vi "CallEdit.vi"(9 "Self Enqueuer":refnum<class "Message Enqueuer.lvclass">, 10 "Configuration":refnum<data-value>, 11 "LogicName":string) -> ()   [LabVIEW 2025, in "PLC_Module.lvlib" / "PLC_Module.lvclass"]
uses:
  PLC_Module.lvclass
  PLC_Data_Config.ctl
  PLC_Data.ctl
  PLC_Data_Type.ctl
  Edit.vi
  PLC_Module.lvclass/PLC_Module.ctl
  <vilib>/ActorFramework/Message Enqueuer/Message Enqueuer.lvclass
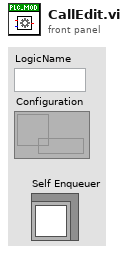
[diagram p1: front panel]
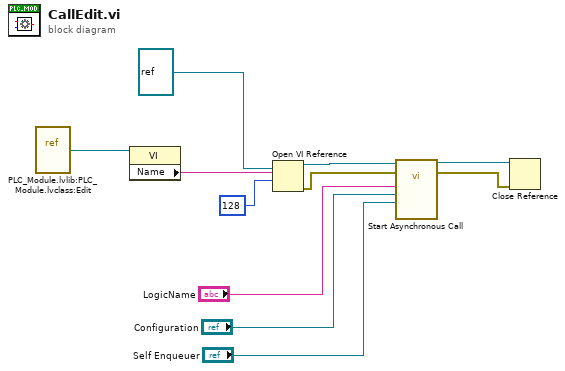
[diagram p0: block diagram]
diagram:
  n1 = vi-ref "PLC_Module.lvlib:PLC_Module.lvclass:Edit.vi"() -> (w11:refnum<vi>)
  n2 = property class="VI"(reference=w11) -> ("Name"=w10:string)  [unwired: 1 in, 2 out]
  n3 = Open VI Reference(type specifier VI Refnum (for type only)=refnum<vi> refnum, vi path=w10, options=128) -> (vi reference=w9:refnum<vi>, error out=w5:errorcluster)  [unwired: 3 in]
  n4 = call-by-ref "Start Asynchronous Call"(reference=w9, error in=w5, "Self Enqueuer"="Self Enqueuer", "Configuration"="Configuration", "LogicName"="LogicName") -> (reference out=w8:refnum<vi>, error out=w4:errorcluster)  [unwired: 9 in]
  n5 = Close Reference(reference=w8, error in (no error)=w4) -> ()  [unwired: 1 out]
